vi "AccessConfigCluster.vi"(3 "error in (no error)":errorcluster, 4 "configuration file path":path, 5 "Action":enum16{"Read", "Write"}(ring)) -> (0 "error out":errorcluster, 1 "error?":bool, 2 "message":string)   [LabVIEW 2012]
uses:
  Config.ctl
  <vilib>/Utility/error.llb/DialogType.ctl
  <vilib>/Utility/config.llb/Read Key (I32).vi
  <vilib>/Utility/config.llb/Read Key (Double).vi
  <vilib>/Utility/config.llb/Write Key (I32).vi
  <vilib>/Utility/config.llb/Write Key (Double).vi
  <vilib>/Utility/config.llb/NI_LVConfig.lvlib
panel:
  in  "ConfigRef":refnum<vi>
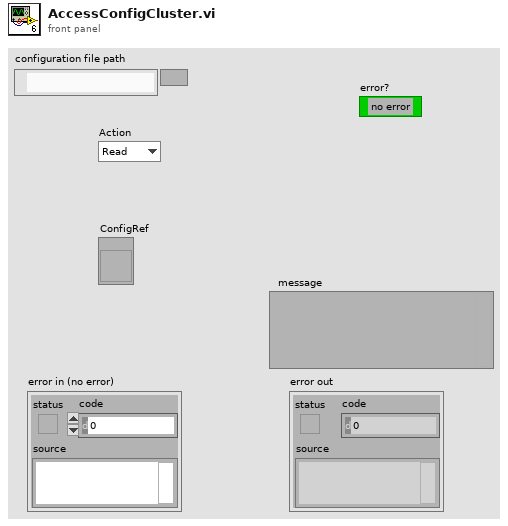
[diagram p1: front panel]
types:
  T1 = typedef "DialogType.ctl" = u16
  T2 = typedef "NI_LVConfig.lvlib/Config Data RefNum.ctl" = refnum<k1>
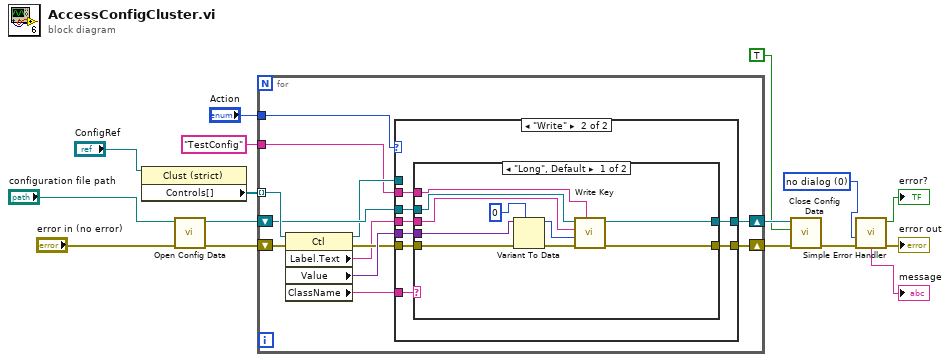
[diagram p0: block diagram]
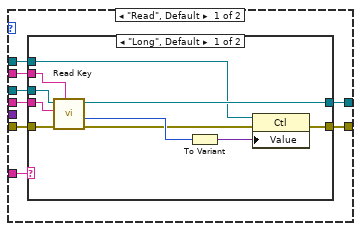
[diagram p2: hidden frame]
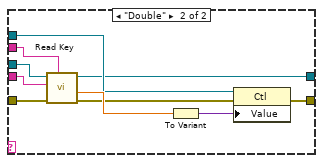
[diagram p3: hidden frame]
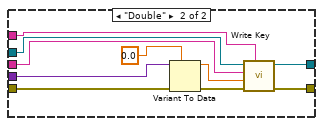
[diagram p4: hidden frame]
diagram:
  w4 = T1 0 items=["no dialog", "OK message", "continue or stop message", "OK message + warnings", "continue/stop + warnings"] ("type of dialog (OK msg:1)")
  n1 = property class="Clust (strict)"(reference="ConfigRef") -> ("Controls[]"=w3:refnum<vi>[])  [unwired: 1 in, 2 out]
  n2 = call <vilib>:"Open Config Data.vi"("error in (no error)"="error in (no error)", "configuration file path"="configuration file path") -> ("error out"=w15:errorcluster, "refnum"=w16:T2)  [unwired: 7 in, 1 out]
  n3 = for {
    tunnel: w3 -> [w28] mode=indexing
    shift-right: [w23] -> w12
    shift-left: w15 -> [w24]
    shift-right: [w22] -> w14
    shift-left: w16 -> [w25]
    tunnel: "Action" -> [w21]
    tunnel: "TestConfig" ("section") -> [w19]
    n4 = property class="Ctl"(reference=w28, error in=w24) -> (reference out=w20:refnum<vi>, error out=w26:errorcluster, "Label.Text"=w17:string, "Value"=w27:variant, "ClassName"=w18:string)
    n5 = case shown="\"Write\"" w21 {
      tunnel: w27 -> [_ w64]
      tunnel: w26 -> [w35 w63]
      tunnel: w25 -> [w36 w62]
      tunnel: [w33 w61] -> w23
      tunnel: [w32 w60] -> w22
      tunnel: w20 -> [w34 _]
      tunnel: w19 -> [w30 w59]
      tunnel: w18 -> [w31 w58]
      tunnel: w17 -> [w29 w57]
      frame "Read", Default {
        n6 = case shown="\"Long\", Default" w31 {
          tunnel: [w39 w49] -> w33
          tunnel: [w44 w50] -> w32
          tunnel: w36 -> [w46 w53]
          tunnel: w35 -> [w45 w51]
          tunnel: w34 -> [w41 w52]
          tunnel: w30 -> [w38 w48]
          tunnel: w29 -> [w37 w47]
          frame "Long", Default {
            n7 = call-poly <vilib>:"Read Key.vi"("section"=w38, "error in (no error)"=w45, "key"=w37, "refnum"=w46) -> ("error out"=w40:errorcluster, "value"=w42:i32, "refnum out"=w44:T2)  [unwired: 1 in, 4 out]
            n8 = To Variant(anything=w42) -> (Variant=w43:variant)
            n9 = property class="Ctl"(reference=w41, error in=w40, "Value"=w43) -> (error out=w39:errorcluster)  [unwired: 1 out]
          }
          frame "Double" {
            n10 = call-poly <vilib>:"Read Key.vi"("section"=w48, "error in (no error)"=w51, "key"=w47, "refnum"=w53) -> ("error out"=w54:errorcluster, "value"=w55:dbl, "refnum out"=w50:T2)  [unwired: 1 in, 4 out]
            n11 = To Variant(anything=w55) -> (Variant=w56:variant)
            n12 = property class="Ctl"(reference=w52, error in=w54, "Value"=w56) -> (error out=w49:errorcluster)  [unwired: 1 out]
          }
        }
      }
      frame "Write" {
        n13 = case shown="\"Long\", Default" w58 {
          tunnel: w64 -> [w74 w83]
          tunnel: w63 -> [w72 w82]
          tunnel: [w69 w78] -> w61
          tunnel: w62 -> [w68 w79]
          tunnel: [w67 w77] -> w60
          tunnel: w59 -> [w66 w76]
          tunnel: w57 -> [w65 w75]
          frame "Long", Default {
            n14 = Variant To Data(error in=w72, type=0, Variant=w74) -> (data=w71:i32, error out=w70:errorcluster)
            n15 = call-poly <vilib>:"Write Key.vi"("section"=w66, "error in (no error)"=w70, "value"=w71, "key"=w65, "refnum"=w68) -> ("error out"=w69:errorcluster, "refnum out"=w67:T2)  [unwired: 4 in, 1 out]
          }
          frame "Double" {
            n16 = Variant To Data(error in=w82, type=0.0, Variant=w83) -> (data=w81:dbl, error out=w80:errorcluster)
            n17 = call-poly <vilib>:"Write Key.vi"("section"=w76, "error in (no error)"=w80, "value"=w81, "key"=w75, "refnum"=w79) -> ("error out"=w78:errorcluster, "refnum out"=w77:T2)  [unwired: 4 in, 1 out]
          }
        }
      }
    }
  }
  n18 = call <vilib>:"Close Config Data.vi"("error in (no error)"=w12, "write file if changed (T)"=TRUE, "refnum"=w14) -> ("error out"=w8:errorcluster)  [unwired: 8 out]
  n19 = call <vilib>:"Simple Error Handler.vi"("type of dialog (OK msg:1)"=w4, "error in (no error)"=w8) -> ("error?"=→"error?":bool, "error out"=→"error out":errorcluster, "message"=→"message":string)  [unwired: 3 in, 2 out]
